vi "My_Test.vi"() -> ()   [LabVIEW 2019]
doc: "Demonstrates the use of the <B>OPC UA Alarms and Conditions</B> functionality as an OPC UA Client."
uses:
  <vilib>/OPCUA/controls/Write Variant Request.ctl
  <vilib>/OPCUA/controls/NodeId.ctl
  <vilib>/OPCUA/controls/Write Status.ctl
  <vilib>/OPCUA/client/Multiple Write Variant.vi
  <vilib>/OPCUA/controls/Subscription Data Change.ctl
  <vilib>/OPCUA/controls/Data Type.ctl
  <vilib>/OPCUA/controls/OPC UA StatusCode.ctl
  <vilib>/OPCUA/NI OPC UA Client.lvlib
panel:
  in  "auto acknowledge":bool
  in  "events view":T1(tab)
  in  "events":i32(listbox)=-1
  in  "acknowledge":bool
  in  "alarms":i32(listbox)=-1
  in  "confirm":bool
  in  "notifier node ID":string="ns=7;s=S71500Fork.3Fork.dbAlarmDevice.Device[1].bAlarmError3"
  in  "start time":timestamp
  in  "history events":i32(listbox)=-1
  in  "end time":timestamp
  in  "history event read":bool
  in  "stop":bool
  in  "server endpoint URL":string="opc.tcp://INOCS:55101"
  # "Overview: Demonstrates the use of the OPC UA Alarms  functionality as an OPC UA Client.\nRequirements: \n1. LabVIEW OPC UA Toolkit\n2. Run this VI on RT targets or Windows\nInstructions:\n1. Specify the server endpoint URL generated by the server.\n2. Run the VI.\n3. Click the auto acknowledge and confirm to choose whether this VI automatically acknowledges the condition."
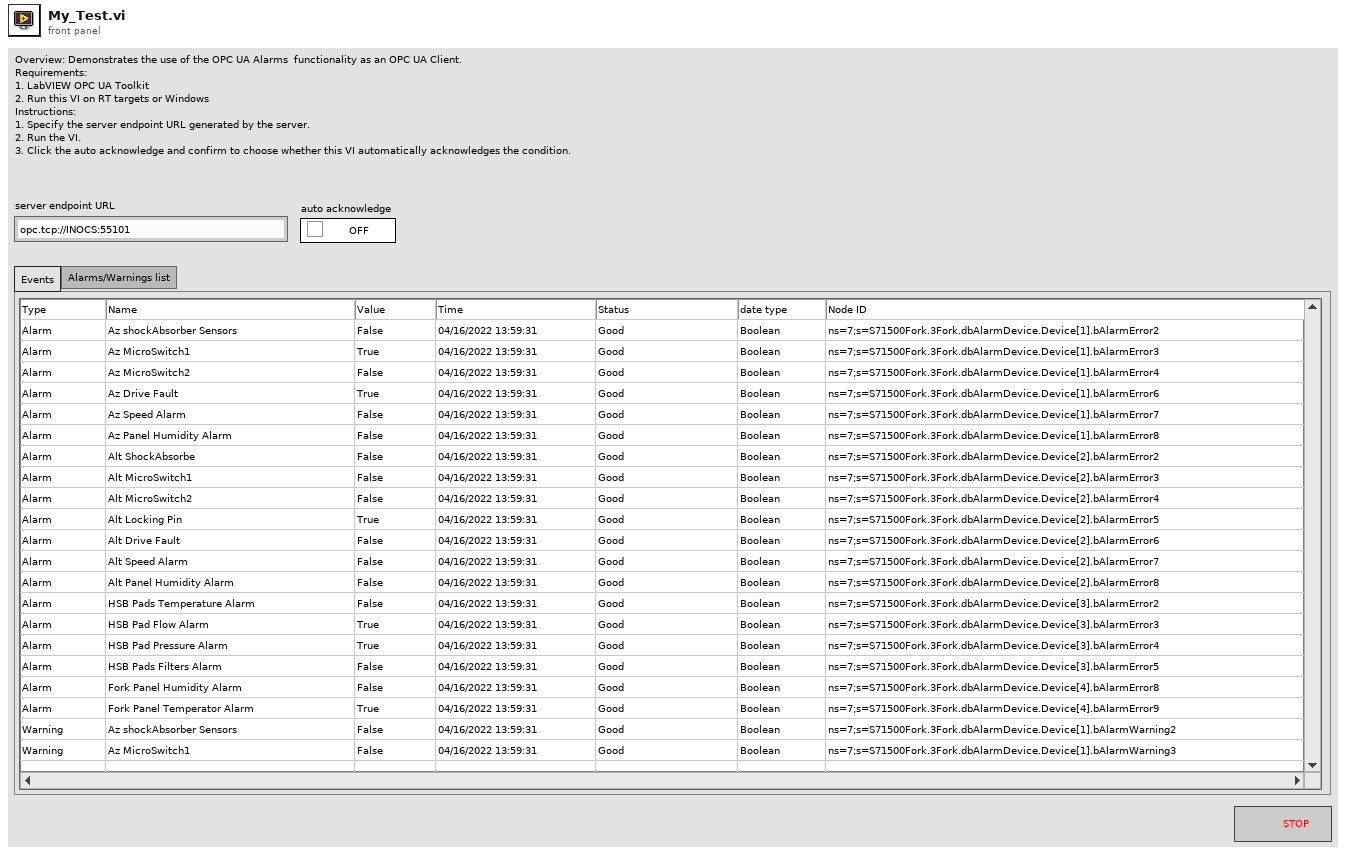
[diagram p1: front panel]
types:
  T1 = enum32{"Events", "Alarms/Warnings list", "History Events"}
  T2 = typedef "OPC UA Client Refnum.ctl" = refnum<k21>
  T3 = typedef "Subscription ID.ctl" = u32
  T4 = typedef "Write Variant Request.ctl" = cluster{"node ID":T5, "value":variant, "timestamp (current time)":timestamp, "node status":T6}
  T5 = typedef "NodeId.ctl" = string
  T6 = typedef "Write Status.ctl" = u32
  T7 = cluster{"start time":timestamp, "end time":timestamp, "num values per node":u32, "return bounds":bool}
  T8 = cluster{"continuation point":variant, "has continuation point?":bool}[]
  T9 = typedef "Subscription Data Change.ctl" = cluster{"node ID":T5, " value":variant, "timestamp":timestamp, "data type":T10, "status code":T11}
  T10 = typedef "Data Type.ctl" = u16
  T11 = typedef "OPC UA StatusCode.ctl" = u32
  T12 = typedef "History Data Result.ctl" = cluster{"node ID":T5, "history data":T13[], "status":T11}
  T13 = typedef "History Data.ctl" = cluster{"value ":variant, "timestamp":timestamp, "node status":T11}
  T14 = cluster{"continuation point":variant, "has continuation point?":bool}
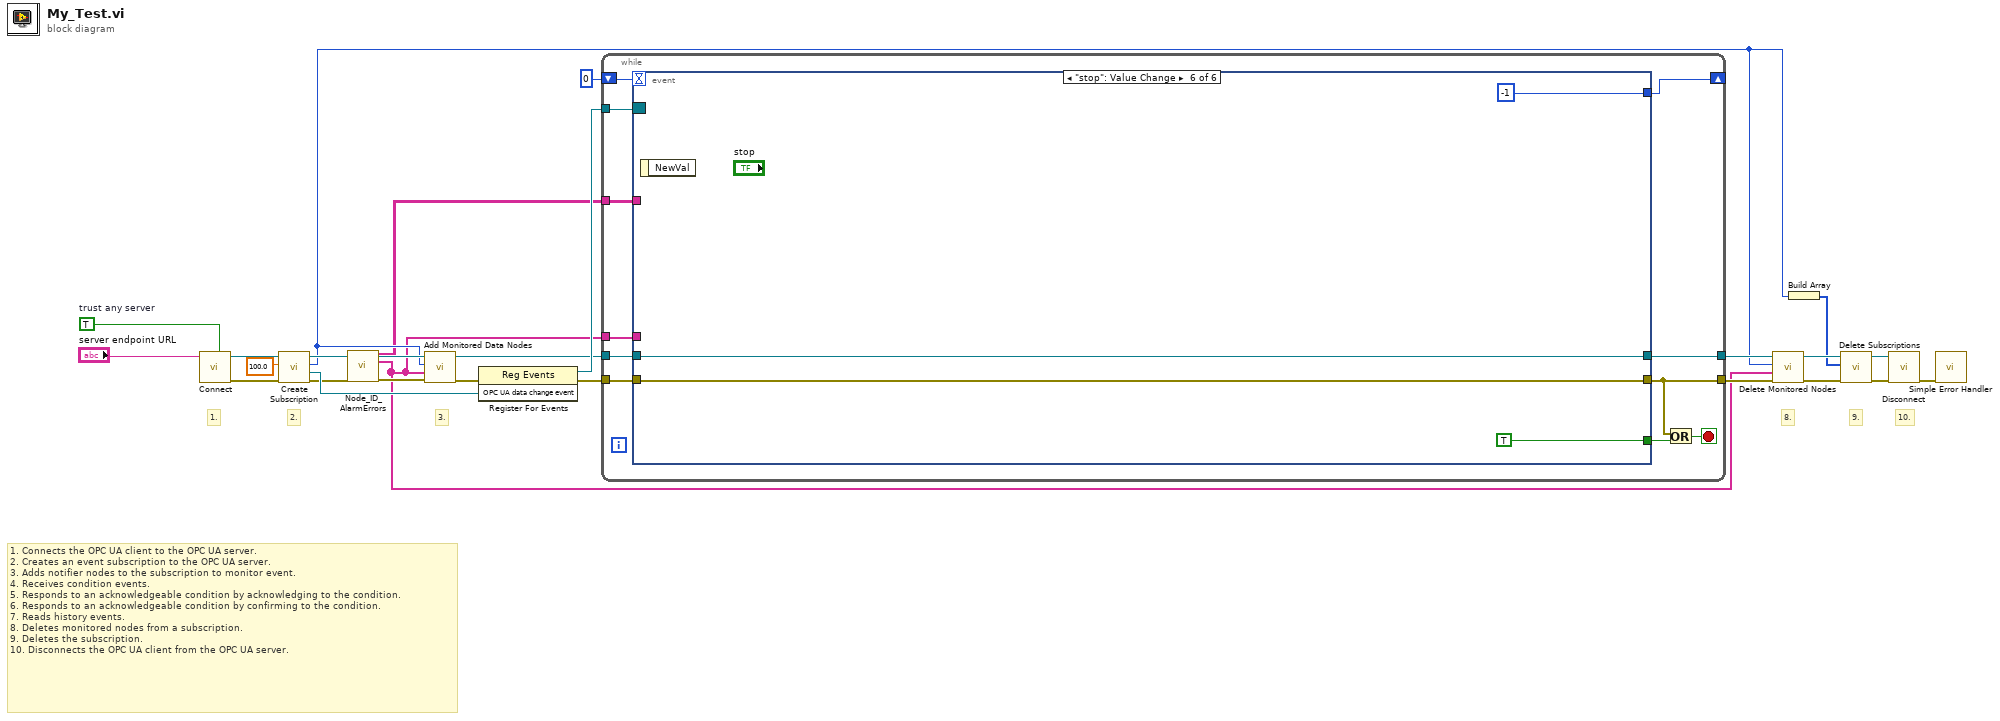
[diagram p0: block diagram]
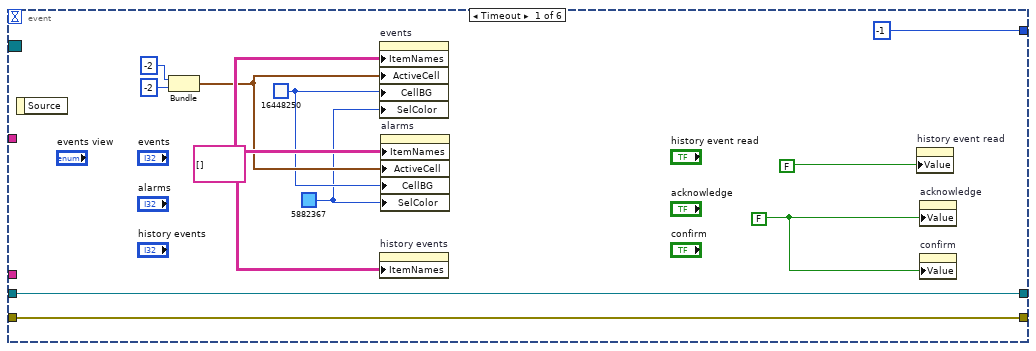
[diagram p2: hidden frame]
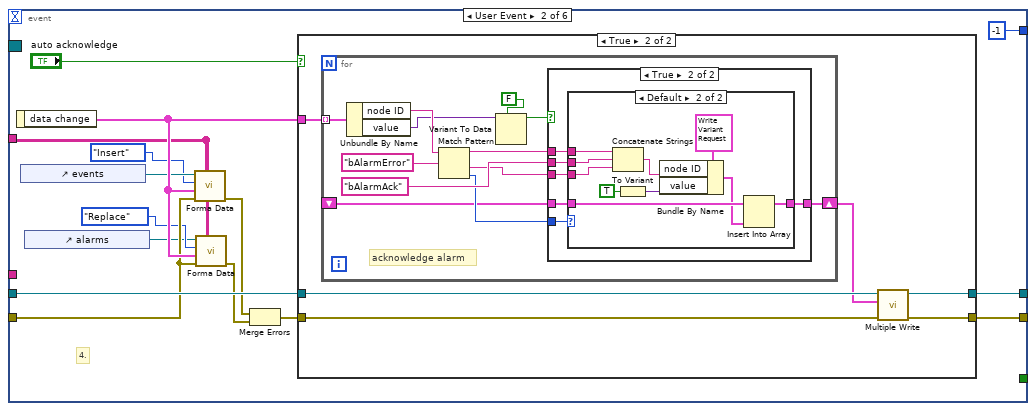
[diagram p3: hidden frame]
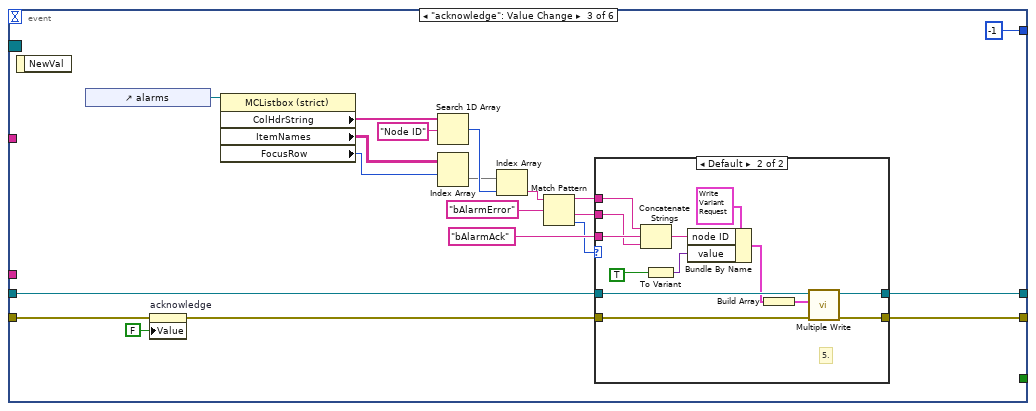
[diagram p7: hidden frame]
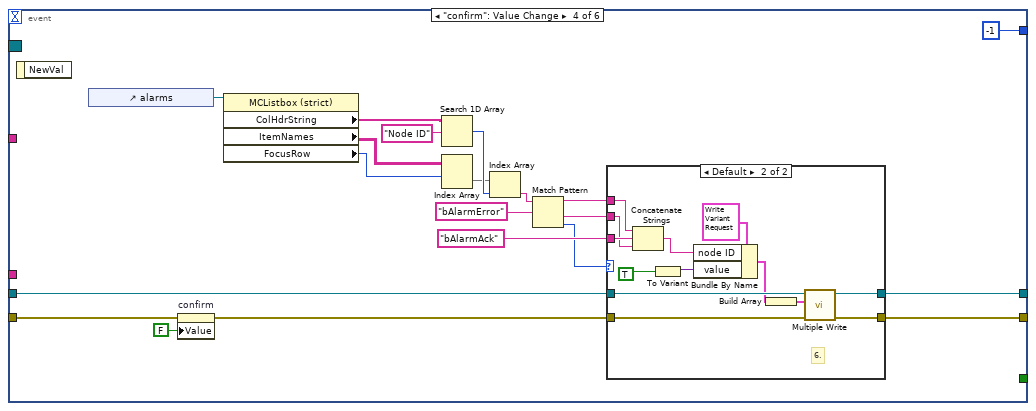
[diagram p9: hidden frame]
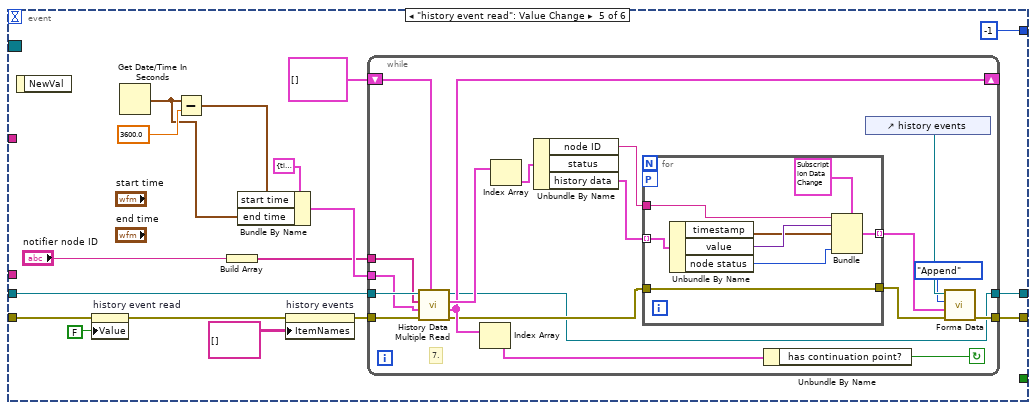
[diagram p11: hidden frame]
diagram:
  w7 = TRUE  # trust any server
  # "9."
  # "8."
  # "10."
  # "3."
  # "2."
  # "1."
  # "1. Connects the OPC UA client to the OPC UA server. \n2. Creates an event subscription to the OPC UA server.\n3. Adds notifier nodes to the subscription to monitor event.\n4. Receives condition events.\n5. Responds to an acknowledgeable condition by acknowledging to the condition. \n6. Responds to an acknowledgeable condition by confirming to the condition. \n7. Reads history events. \n8. Deletes monitored nodes from a subscription.\n9. Deletes the subscription. \n10. Disconnects the OPC UA client from the OPC UA server."
  n1 = call <vilib>:"Connect.vi"("trust any server (F)"=w7, "server endpoint URL"="server endpoint URL") -> ("error out"=w22:errorcluster, "OPC UA client refnum out"=w21:T2)  [unwired: 7 in, 1 out]
  n2 = call <vilib>:"Create Subscription.vi"("error in (no error)"=w22, "publishing interval (1000 ms)"=100.0 ("update rate (1000 ms)"), "OPC UA client refnum in"=w21) -> ("error out"=w5:errorcluster, "OPC UA data change event"=w6:refnum<user-event>, "subscription ID out"=w3:T3, "OPC UA client refnum out"=w25:T2)  [unwired: 4 in, 1 out]
  n3 = call "Node_ID_AlarmErrors.vi"("error in"=w5) -> ("transposed array"=w2:string[][], "Node ID"=w1:string[], "error out"=w4:errorcluster)  [unwired: 8 in, 4 out]
  n4 = call <vilib>:"Add Monitored Data Nodes.vi"("error in (no error)"=w4, "node IDs"=w1, "subscription ID in"=w3, "OPC UA client refnum in"=w25) -> ("error out"=w24:errorcluster, "OPC UA client refnum out"=w17:T2)  [unwired: 4 in, 2 out]
  n5 = register-events(error in=w24, w6) -> (reference out=w19:refnum<event-registration>, error out=w18:errorcluster)  [unwired: 1 in]
  n6 = while {
    tunnel: w19 -> [w36]
    tunnel: w18 -> [w35]
    tunnel: [w29] -> w15
    tunnel: w17 -> [w34]
    tunnel: [w33] -> w16
    shift-right: [w31] -> _
    shift-left: 0 -> [w32]
    tunnel: w2 -> [w27]
    tunnel: w1 -> [w26]
    stop <- w28 stop-if-true
    n7 = event shown="[5] \"stop\": Value Change" {
      selector: w36 -> [_ _ _ _ _ _]
      dyn-events: _ -> [_ _ _ _ _ _]
      timeout: w32 -> [_ _ _ _ _ _]
      tunnel: w35 -> [w43 w55 w109 w151 w179 w217]
      tunnel: [w43 w60 w111 w149 w177 w217] -> w29
      tunnel: w34 -> [w44 w62 w110 w152 w180 w218]
      tunnel: [w44 w61 w112 w150 w178 w218] -> w33
      tunnel: [-1 -1 -1 -1 -1 -1] -> w31
      tunnel: [_ _ _ _ _ TRUE] -> w30
      tunnel: w27 -> [_ w48 _ _ _ _]
      tunnel: w26 -> [_ _ _ _ _ _]
      event Timeout {
        w37 = u32 5882367 ("Selection Color")
        w38 = u32 16448250 ("Active Cell:Cell Background Color")
        w46 = FALSE
        w47 = string[][] [] ("Item Names")
        n8 = event-data() -> ()  [unwired: 1 in, 1 out]
        n9 = Bundle(-2, -2) -> (w39:cluster{i32, i32})  [unwired: 1 in]
        n10 = property on="events" class="MCListbox (strict)"("ItemNames"=w47, "ActiveCell"=w39, "CellBG"=w38, "SelColor"=w37) -> ()  [unwired: 2 in, 2 out]
        n11 = property on="history events" class="MCListbox (strict)"("ItemNames"=w47) -> ()  [unwired: 2 in, 2 out]
        n12 = property on="alarms" class="MCListbox (strict)"("ItemNames"=w47, "ActiveCell"=w39, "CellBG"=w38, "SelColor"=w37) -> ()  [unwired: 2 in, 2 out]
        n13 = property on="history event read" class="Bool (strict)"("Value"=FALSE) -> ()  [unwired: 2 in, 2 out]
        n14 = property on="acknowledge" class="Bool (strict)"("Value"=w46) -> ()  [unwired: 2 in, 2 out]
        n15 = property on="confirm" class="Bool (strict)"("Value"=w46) -> ()  [unwired: 2 in, 2 out]
      }
      event User Event {
        # "4."
        n16 = event-data() -> ("data change"=w58:T9[])  [unwired: 1 in]
        n17 = control-ref of="events"() -> (w53:refnum<vi>)
        n18 = control-ref of="alarms"() -> (w51:refnum<vi>)
        n19 = call "Forma Data.vi"("appended array"=w48, "error in"=w55, "data array"=w58, "type"=enum16{"Insert", "Replace", "Append"}."Insert", "Multicolumn Listbox"=w53) -> ("error out"=w50:errorcluster)  [unwired: 3 in, 3 out]
        n20 = call "Forma Data.vi"("appended array"=w48, "error in"=w55, "data array"=w58, "type"=enum16{"Insert", "Replace", "Append"}."Replace", "Multicolumn Listbox"=w51) -> ("error out"=w49:errorcluster)  [unwired: 3 in, 3 out]
        n21 = Merge Errors(w50, w49) -> (w56:errorcluster)
        n22 = case shown="True" "auto acknowledge" {
          tunnel: w58 -> [_ w70]
          tunnel: w62 -> [w64 w68]
          tunnel: w56 -> [w63 w69]
          tunnel: [w64 w66] -> w61
          tunnel: [w63 w67] -> w60
          frame False {
          }
          frame True {
            n23 = for {
              tunnel: w70 -> [w82] mode=indexing
              shift-right: [w81] -> w65
              shift-left: _ -> [w74]
              # "acknowledge alarm"
              n24 = Unbundle By Name(w82) -> ("node ID"=w79:T5, "value"=w72:variant)
              n25 = Match Pattern(string=w79, regular expression="bAlarmError" ("search string/char (-)")) -> (before substring=w78:T5, after substring=w76:T5, offset past match=w75:i32)  [unwired: 1 in, 1 out]
              n26 = Variant To Data(type=FALSE, Variant=w72) -> (data=w71:bool)  [unwired: 1 in, 1 out]
              n27 = case shown="True" w71 {
                tunnel: [w83 w89] -> w81
                tunnel: w78 -> [_ w88]
                tunnel: "bAlarmAck" ("string") -> [_ w87]
                tunnel: w76 -> [_ w86]
                tunnel: w75 -> [_ w85]
                tunnel: w74 -> [w83 w84]
                frame False {
                }
                frame True {
                  n28 = case shown="Default" w85 {
                    tunnel: [w90 w91] -> w89
                    tunnel: w88 -> [_ w96]
                    tunnel: w87 -> [_ w95]
                    tunnel: w86 -> [_ w94]
                    tunnel: w84 -> [w90 w93]
                    frame -1 {
                    }
                    frame Default {
                      n29 = Concatenate Strings(w96, w95, w94) -> (w97:string)
                      n30 = To Variant(anything=TRUE) -> (Variant=w98:variant)
                      n31 = Bundle By Name(cluster=T4 {"node ID"="", "value"=variant, "timestamp (current time)"=timestamp(0 s since 1904-01-01), "node status"=0} ("requests"), "node ID"=w97, "value"=w98) -> (w92:T4)
                      n32 = Insert Into Array(array=w93, new element=w92) -> (w91:T4[])  [unwired: 1 in]
                    }
                  }
                }
              }
            }
            n33 = call-poly <vilib>:"Multiple Write.vi"("error in (no error)"=w69, "requests"=w65, "OPC UA client refnum in"=w68) -> ("error out"=w67:errorcluster, "OPC UA client refnum out"=w66:T2)  [unwired: 5 in, 2 out]
          }
        }
      }
      event "acknowledge": Value Change {
        n34 = event-data() -> ()  [unwired: 1 in, 1 out]
        n35 = control-ref of="alarms"() -> (w120:refnum<vi>)
        n36 = property on="acknowledge" class="Bool (strict)"(error in=w109, "Value"=FALSE ("acknowledge")) -> (error out=w114:errorcluster)  [unwired: 1 in, 1 out]
        n37 = property class="MCListbox (strict)"(reference=w120) -> ("ColHdrString"=w107:string[], "ItemNames"=w119:string[][], "FocusRow"=w118:i32)  [unwired: 1 in, 2 out]
        n38 = Search 1D Array(1D array=w107, element="Node ID") -> (index of element=w116:i32)  [unwired: 1 in]
        n39 = Index Array(array=w119, index (row)=w118) -> (element=w115:string[])  [unwired: 1 in]
        n40 = Index Array(array=w115, index=w116) -> (element=w106:string)
        n41 = Match Pattern(string=w106, regular expression="bAlarmError" ("search string/char (-)")) -> (before substring=w104:string, after substring=w102:string, offset past match=w101:i32)  [unwired: 1 in, 1 out]
        n42 = case shown="Default" w101 {
          tunnel: w114 -> [w121 w135]
          tunnel: [w122 w134] -> w112
          tunnel: [w121 w133] -> w111
          tunnel: w110 -> [w122 w132]
          tunnel: w104 -> [_ w126]
          tunnel: "bAlarmAck" ("string") -> [_ w125]
          tunnel: w102 -> [_ w124]
          frame -1 {
          }
          frame Default {
            # "5."
            n43 = Concatenate Strings(w126, w125, w124) -> (w123:string)
            n44 = To Variant(anything=TRUE) -> (Variant=w129:variant)
            n45 = Bundle By Name(cluster=T4 {"node ID"="", "value"=variant, "timestamp (current time)"=timestamp(0 s since 1904-01-01), "node status"=0} ("request"), "node ID"=w123, "value"=w129) -> (w131:T4)
            n46 = Build Array(w131) -> (w127:T4[])
            n47 = call-poly <vilib>:"Multiple Write.vi"("error in (no error)"=w135, "requests"=w127, "OPC UA client refnum in"=w132) -> ("error out"=w133:errorcluster, "OPC UA client refnum out"=w134:T2)  [unwired: 5 in, 2 out]
          }
        }
      }
      event "confirm": Value Change {
        n48 = event-data() -> ()  [unwired: 1 in, 1 out]
        n49 = control-ref of="alarms"() -> (w155:refnum<vi>)
        n50 = property on="confirm" class="Bool (strict)"(error in=w151, "Value"=FALSE ("confirm")) -> (error out=w153:errorcluster)  [unwired: 1 in, 1 out]
        n51 = property class="MCListbox (strict)"(reference=w155) -> ("ColHdrString"=w137:string[], "ItemNames"=w138:string[][], "FocusRow"=w139:i32)  [unwired: 1 in, 2 out]
        n52 = Search 1D Array(1D array=w137, element="Node ID") -> (index of element=w146:i32)  [unwired: 1 in]
        n53 = Index Array(array=w138, index (row)=w139) -> (element=w145:string[])  [unwired: 1 in]
        n54 = Index Array(array=w145, index=w146) -> (element=w144:string)
        n55 = Match Pattern(string=w144, regular expression="bAlarmError" ("search string/char (-)")) -> (before substring=w142:string, after substring=w140:string, offset past match=w136:i32)  [unwired: 1 in, 1 out]
        n56 = case shown="Default" w136 {
          tunnel: w153 -> [w156 w170]
          tunnel: w152 -> [w157 w169]
          tunnel: [w157 w168] -> w150
          tunnel: [w156 w167] -> w149
          tunnel: w142 -> [_ w161]
          tunnel: "bAlarmAck" ("string") -> [_ w160]
          tunnel: w140 -> [_ w159]
          frame -1 {
          }
          frame Default {
            # "6."
            n57 = Concatenate Strings(w161, w160, w159) -> (w158:string)
            n58 = To Variant(anything=TRUE) -> (Variant=w164:variant)
            n59 = Bundle By Name(cluster=T4 {"node ID"="", "value"=variant, "timestamp (current time)"=timestamp(0 s since 1904-01-01), "node status"=0} ("request"), "node ID"=w158, "value"=w164) -> (w166:T4)
            n60 = Build Array(w166) -> (w163:T4[])
            n61 = call-poly <vilib>:"Multiple Write.vi"("error in (no error)"=w170, "requests"=w163, "OPC UA client refnum in"=w169) -> ("error out"=w167:errorcluster, "OPC UA client refnum out"=w168:T2)  [unwired: 5 in, 2 out]
          }
        }
      }
      event "history event read": Value Change {
        n62 = event-data() -> ()  [unwired: 1 in, 1 out]
        n63 = property on="history event read" class="Bool (strict)"(error in=w179, "Value"=FALSE) -> (error out=w181:errorcluster)  [unwired: 1 in, 1 out]
        n64 = Get Date/Time In Seconds() -> (seconds since 1Jan1904=w173:timestamp)
        n65 = Subtract(x=w173, y=3600.0 ("time span")) -> (x-y=w174:timestamp)
        n66 = Build Array("notifier node ID") -> (w172:string[])
        n67 = Bundle By Name(cluster=T7 {"start time"=timestamp(0 s since 1904-01-01), "end time"=timestamp(0 s since 1904-01-01), "num values per node"=0, "return bounds"=FALSE} ("request"), "start time"=w174, "end time"=w173) -> (w185:T7)
        n68 = property on="history events" class="MCListbox (strict)"(error in=w181, "ItemNames"=string[][] [] ("Item Names")) -> (error out=w184:errorcluster)  [unwired: 1 in, 1 out]
        n69 = while {
          tunnel: w172 -> [w198]
          tunnel: w185 -> [w188]
          tunnel: [w192] -> w178
          tunnel: [w193] -> w177
          shift-right: [w201] -> _
          shift-left: T8 [] ("continuation points in") -> [w202]
          tunnel: w184 -> [w200]
          tunnel: w180 -> [w199]
          stop <- w203 continue-if-true
          # "7."
          n70 = call <vilib>:"History Data Multiple Read.vi"("continuation points in"=w202, "error in (no error)"=w200, "request"=w188, "node IDs"=w198, "OPC UA client refnum in"=w199) -> ("error out"=w195:errorcluster, "continuation points out"=w201:T8, "results"=w206:T12[], "OPC UA client refnum out"=w192:T2)  [unwired: 2 in, 1 out]
          n71 = Index Array(array=w201) -> (element=w204:T14)  [unwired: 1 in]
          n72 = Index Array(array=w206) -> (element=w205:T12)  [unwired: 1 in]
          n73 = Unbundle By Name(w205) -> ("node ID"=w196:T5, "history data"=w197:T13[])  [unwired: 1 out]
          n74 = for {
            tunnel: w197 -> [w214] mode=indexing
            tunnel: [w213] -> w189 mode=indexing
            tunnel: w195 -> [w208]
            tunnel: [w208] -> w194
            workers-P: _ -> [_]
            tunnel: w196 -> [w207]
            n75 = Unbundle By Name(w214) -> ("timestamp"=w210:timestamp, "value"=w211:variant, "node status"=w209:T11)
            n76 = Bundle(cluster=T9 {"node ID"="", " value"=variant, "timestamp"=timestamp(0 s since 1904-01-01), "data type"=0, "status code"=0} ("data array"), "node ID"=w207, "value"=w211, "timestamp"=w210, "status code"=w209) -> (w213:T9)  [unwired: 1 in]
          }
          n77 = Unbundle By Name(w204) -> ("has continuation point?"=w203:bool)
          n78 = control-ref of="history events"() -> (w191:refnum<vi>)
          n79 = call "Forma Data.vi"("error in"=w194, "data array"=w189, "type"=enum16{"Insert", "Replace", "Append"}."Append", "Multicolumn Listbox"=w191) -> ("error out"=w193:errorcluster)  [unwired: 4 in, 3 out]
        }
      }
      event "stop": Value Change {
        n80 = event-data() -> ()  [unwired: 1 in, 1 out]
      }
    }
    n81 = Or(x=w29, y=w30) -> (x .or. y?=w28:bool)
  }
  n82 = call <vilib>:"Delete Monitored Nodes.vi"("error in (no error)"=w15, "node IDs"=w1, "subscription ID in"=w3, "OPC UA client refnum in"=w16) -> ("error out"=w13:errorcluster, "OPC UA client refnum out"=w14:T2)  [unwired: 3 in, 3 out]
  n83 = Build Array(w3) -> (w11:T3[])
  n84 = call <vilib>:"Delete Subscriptions.vi"("error in (no error)"=w13, "subscription IDs"=w11, "OPC UA client refnum in"=w14) -> ("error out"=w9:errorcluster, "OPC UA client refnum out"=w12:T2)  [unwired: 6 in, 1 out]
  n85 = call <vilib>:"Disconnect.vi"("error in (no error)"=w9, "OPC UA client refnum in"=w12) -> ("error out"=w8:errorcluster)  [unwired: 9 in]
  n86 = call <vilib>:"Simple Error Handler.vi"("error in (no error)"=w8) -> ()  [unwired: 4 in, 5 out]
